vi "Calculate Checksum.vi"(6 "error in (no error)":errorcluster, 9 "string":string) -> (0 "error out":errorcluster, 3 "checksum":string)   [LabVIEW 2017, in "NMEA API.lvlib"]
doc: "This VI takes a string and calculates the NMEA checksum. The string should be all of the characters between the sentence start character '$' and the sentence termination character '*'. The checksum is the xor sum of every byte of XXX in 2 hex characters."
uses:
  <vilib>/robotics/Protocols/NMEA/NMEA API.lvlib
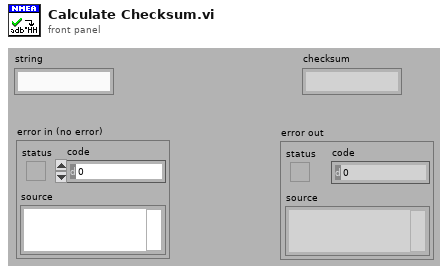
[diagram p1: front panel]
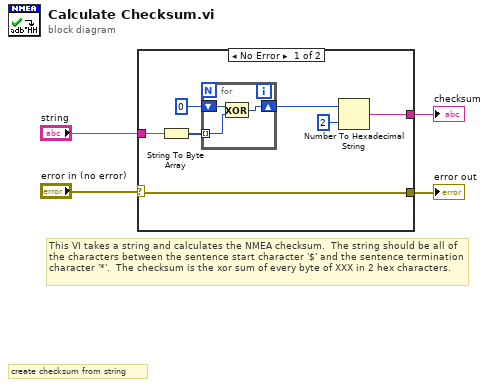
[diagram p0: block diagram]
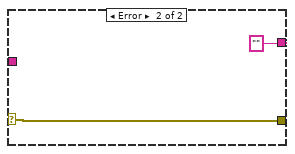
[diagram p2: hidden frame]
diagram:
  # "This VI takes a string and calculates the NMEA checksum.  The string should be all of the characters between the sentence start character '$' and the sentence termination character '*'.  The checksum is the xor sum of every byte of XXX in 2 hex characters."
  # "create checksum from string"
  n1 = case shown="No Error" "error in (no error)" {
    selector: "error in (no error)" -> [w6 w16]
    tunnel: "string" -> [w7 _]
    tunnel: [w6 w16] -> w2
    tunnel: [w8 ""] -> w1
    frame No Error {
      n2 = String To Byte Array(string=w7) -> (unsigned byte array=w11:u8[])
      n3 = for {
        tunnel: w11 -> [w14] mode=indexing
        shift-right: [w12] -> w9
        shift-left: u8 0 -> [w13]
        n4 = Exclusive Or(1:w14, 2:w13) -> (0:w12:u8)
      }
      n5 = Number To Hexadecimal String(1:i16 2 ("width (-)"), 2:w9) -> (0:w8:string)
    }
    frame Error {
    }
  }
  "checksum" <- w1
  "error out" <- w2
